vi "Logistic_Regression_with_iris_data.vi"() -> ()   [LabVIEW 2020]
doc: "Using logistic regression to classify the iris dataset."
uses:
  Model/Supervised/Linear_model/LinearClassifiers/LogisticRegression/Controls/logistic_regression_params.ctl
  Model/Supervised/Linear_model/LinearClassifiers/LogisticRegression/LogisticRegression.lvclass
  C:/Users/cipop/TDF Dropbox/2_Technologies de France/1 - Services et Etudes/PLAIY/2 - DEV/PLAIYLAB/code/Model/Model.lvclass
  Model/Supervised/Linear_model/LinearClassifiers/LogisticRegression/LogisticRegression.vi
panel:
  out "score":dbl
  out "y":dbl[][](array[numeric])
  in  "params":T1={"penalty"="l2", "dual"=FALSE, "tol"=0.0001, "C"=1.0, "fit_intercept"=FALSE, "intercept_scaling"=1.0, "class_weight"={"class_weight_type"="None", "class_weight_dict"=""}, "random_state"=0.0, "solver"="lbfgs", "max_iter"=100.0, "multi_class"="auto", "verbose"=0.0, "warm_start"=FALSE, "n_jobs"=1.0, "l1_ratio"={"l1_ratio_type"="None", "l1_ratio_float"=0.0}}
  out "XY Graph":T2(graph)
  out "error out":errorcluster
  out "X":dbl[][](array[numeric])
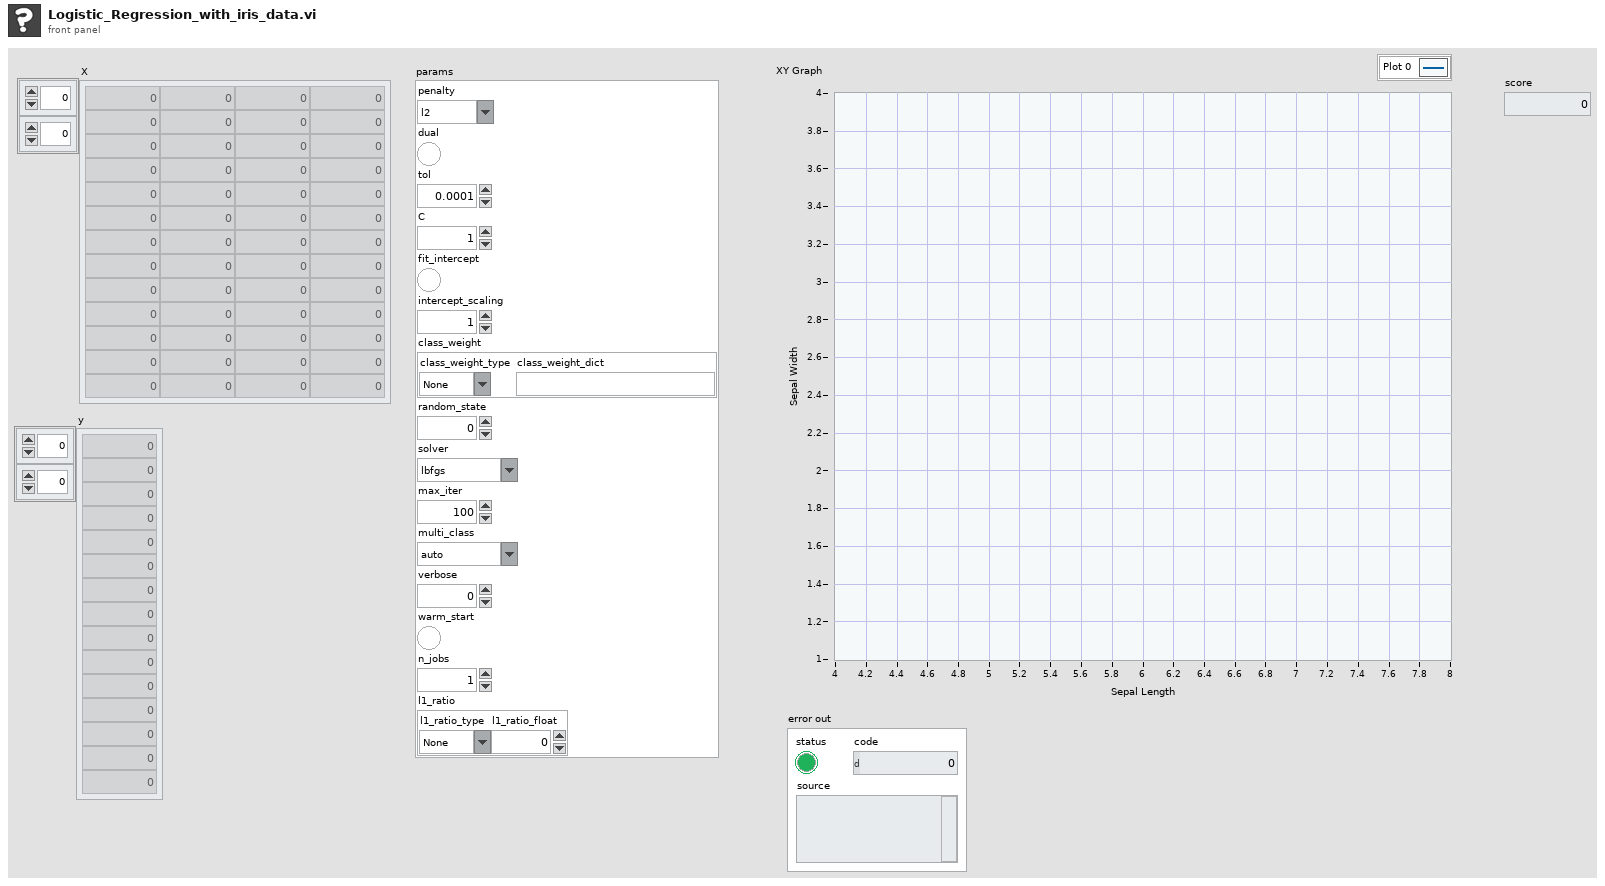
[diagram p1: front panel]
types:
  T1 = typedef "logistic_regression_params.ctl" = cluster{"penalty":string, "dual":bool, "tol":dbl, "C":dbl, "fit_intercept":bool, "intercept_scaling":dbl, "class_weight":cluster{"class_weight_type":string, "class_weight_dict":string}, "random_state":dbl, "solver":string, "max_iter":dbl, "multi_class":string, "verbose":dbl, "warm_start":bool, "n_jobs":dbl, "l1_ratio":cluster{"l1_ratio_type":string, "l1_ratio_float":dbl}}
  T2 = cluster{"XY Graph":cluster{"X":dbl, "Y":dbl}[]}[]
  T3 = cluster{"X Train":dbl[][], "X Test":dbl[][], "Y Train":dbl[][], "Y Test":dbl[][]}
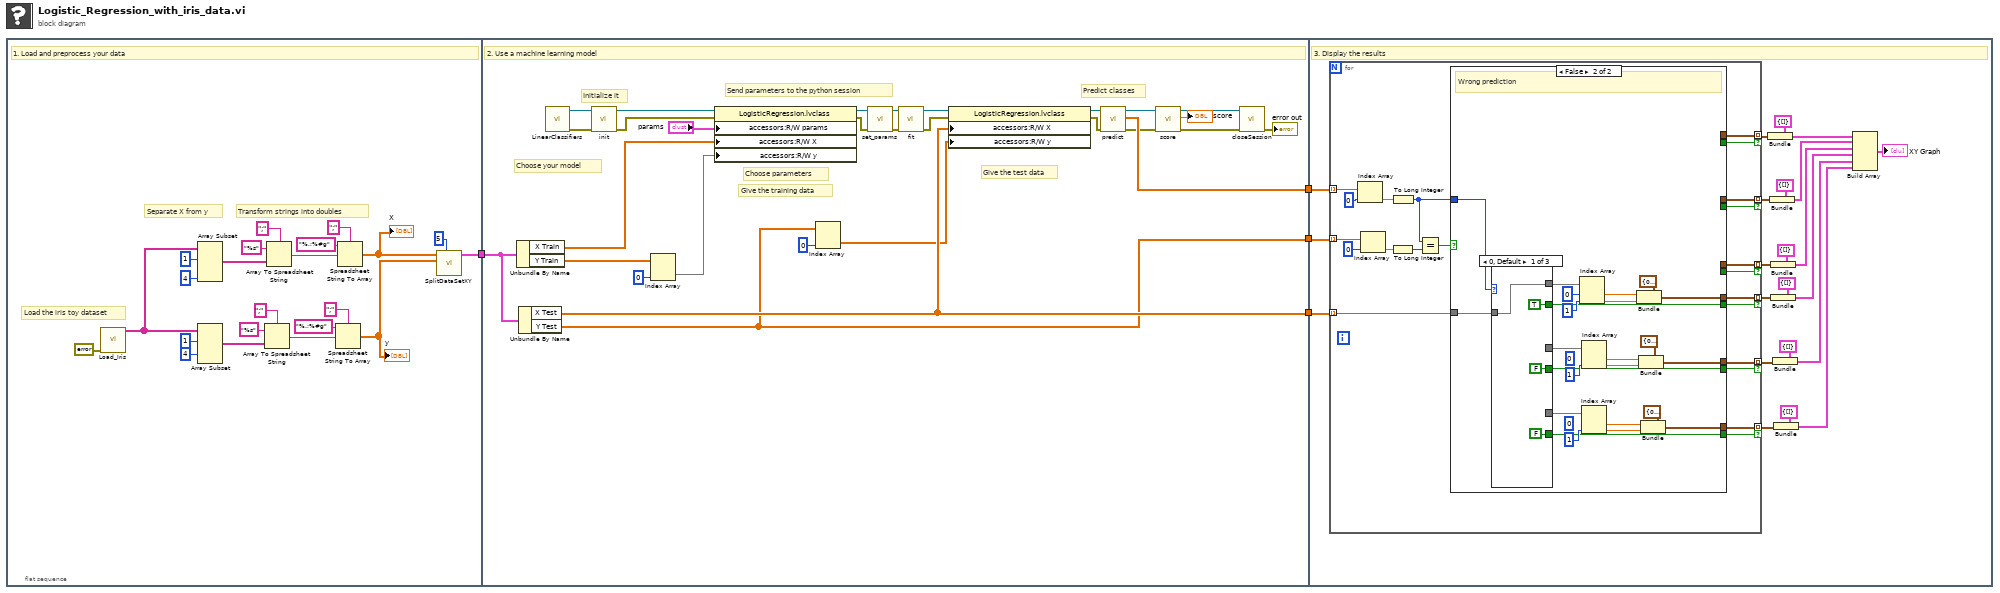
[diagram p0: block diagram]
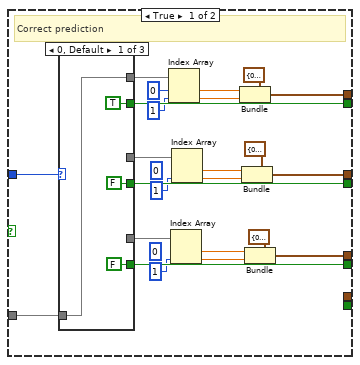
[diagram p2: hidden frame]
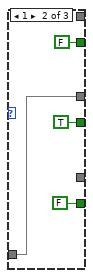
[diagram p3: hidden frame]
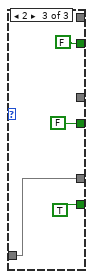
[diagram p4: hidden frame]
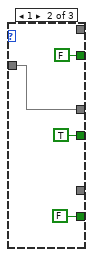
[diagram p5: hidden frame]
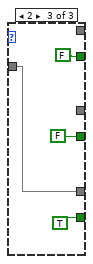
[diagram p6: hidden frame]
diagram:
  n1 = flat-sequence {
    tunnel: [w6] -> w2
    tunnel: [w47] -> w4
    tunnel: [w40] -> w3
    tunnel: w2 -> [w43]
    tunnel: [w33] -> w1
    tunnel: w4 -> [w76]
    tunnel: w3 -> [w77]
    tunnel: w1 -> [w65]
    frame #0 {
      # "Transform strings into doubles"
      # "Separate X from y"
      # "Load the iris toy dataset"
      # "1. Load and preprocess your data"
      n2 = call "Load_Iris.vi"("error in"=errorcluster {"status"=FALSE, "code"=0, "source"=""}) -> ("Tableau"=w21:string[][])  [unwired: 9 in, 1 out]
      n3 = Array Subset(array=w21, index (row)=1 ("index"), length (col)=4 ("length")) -> (w20:string[][])  [unwired: 2 in]
      n4 = Array Subset(array=w21, index (row)=1 ("index"), index (col)=4 ("index")) -> (w9:string[][])  [unwired: 2 in]
      n5 = Array To Spreadsheet String(delimiter (Tab)=";", array=w9, 3:"%s" ("format string")) -> (spreadsheet string=w10:string)
      n6 = Array To Spreadsheet String(delimiter (Tab)=";", array=w20, 3:"%s" ("format string")) -> (spreadsheet string=w15:string)
      n7 = Spreadsheet String To Array(delimiter (Tab)=";", format string="%.;%#g", spreadsheet string=w10) -> (array=w7:dbl[][])  [unwired: 1 in]
      "y" <- w7
      n8 = Spreadsheet String To Array(delimiter (Tab)=";", format string="%.;%#g", spreadsheet string=w15) -> (array=w8:dbl[][])  [unwired: 1 in]
      "X" <- w8
      n9 = call "SplitDataSetXY.vi"("%SplitTrain"=5, "Y"=w7, "X"=w8) -> ("Split"=w6:T3)  [unwired: 7 in, 1 out]
    }
    frame #1 {
      # "Predict classes"
      # "Give the test data"
      # "Send parameters to the python session"
      # "Give the training data"
      # "Choose parameters"
      # "Initialize it"
      # "Choose your model"
      # "2. Use a machine learning model"
      n10 = Unbundle By Name(w43) -> ("X Train"=w46:dbl[][], "Y Train"=w45:dbl[][])
      n11 = Unbundle By Name(w43) -> ("X Test"=w40:dbl[][], "Y Test"=w33:dbl[][])
      n12 = call-poly "LinearClassifiers.vi"() -> ("error out"=w31:errorcluster, "out"=w51:refnum<class "LogisticRegression.lvclass">)  [unwired: 10 in]
      n13 = call-dynamic "init.vi"("error in (no error)"=w31, "Model en entrée"=w51) -> ("error out"=w55:errorcluster, "Model en sortie"=w54:refnum<class "LogisticRegression.lvclass">)  [unwired: 8 in]
      n14 = Index Array(array=w45, index (col)=0 ("disabled index (col)")) -> (element=w44:dbl[])  [unwired: 1 in]
      n15 = property class="LogisticRegression.lvclass"(reference=w54, error in=w55, "accessors:R/W params"="params", "accessors:R/W X"=w46, "accessors:R/W y"=w44) -> (reference out=w53:refnum<class "LogisticRegression.lvclass">, error out=w52:errorcluster)
      n16 = Index Array(array=w33, index (col)=0 ("disabled index (col)")) -> (element=w32:dbl[])  [unwired: 1 in]
      n17 = call-dynamic "set_params.vi"("error in (no error)"=w52, "LogisticRegression.lvclass 2"=w53) -> ("error out"=w48:errorcluster, "LogisticRegression.lvclass"=w49:refnum<class "LogisticRegression.lvclass">)  [unwired: 8 in]
      n18 = call-dynamic "fit.vi"("error in (no error)"=w48, "LogisticRegression.lvclass 2"=w49) -> ("error out"=w41:errorcluster, "LogisticRegression.lvclass"=w42:refnum<class "LogisticRegression.lvclass">)  [unwired: 8 in]
      n19 = property class="LogisticRegression.lvclass"(reference=w42, error in=w41, "accessors:R/W X"=w40, "accessors:R/W y"=w32) -> (reference out=w38:refnum<class "LogisticRegression.lvclass">, error out=w39:errorcluster)
      n20 = call-dynamic "predict.vi"("error in (no error)"=w39, "LogisticRegression.lvclass 2"=w38) -> ("error out"=w35:errorcluster, "C"=w47:dbl[][], "LogisticRegression.lvclass"=w37:refnum<class "LogisticRegression.lvclass">)  [unwired: 7 in]
      n21 = call-dynamic "score.vi"("error in (no error)"=w35, "LogisticRegression.lvclass 2"=w37) -> ("error out"=w30:errorcluster, "score"=→"score":dbl, "LogisticRegression.lvclass"=w36:refnum<class "LogisticRegression.lvclass">)  [unwired: 7 in]
      n22 = call-dynamic "closeSession.vi"("error in"=w30, "Python en entrée"=w36) -> ("error out"=→"error out":errorcluster)  [unwired: 8 in, 1 out]
    }
    frame #2 {
      # "3. Display the results"
      n23 = for {
        tunnel: w77 -> [w96] mode=indexing
        tunnel: w76 -> [w99] mode=indexing
        tunnel: [w92] -> w74 mode=indexing if=w95
        tunnel: [w91] -> w72 mode=indexing if=w94
        tunnel: [w90] -> w70 mode=indexing if=w93
        tunnel: w65 -> [w87] mode=indexing
        tunnel: [w84] -> w61 mode=indexing if=w83
        tunnel: [w82] -> w60 mode=indexing if=w81
        tunnel: [w80] -> w59 mode=indexing if=w79
        n24 = Index Array(array=w99, index=0) -> (element=w97:dbl)
        n25 = Index Array(array=w87, index=0) -> (element=w88:dbl)
        n26 = To Long Integer(number=w88) -> (32bit integer=w85:i32)
        n27 = To Long Integer(number=w97) -> (32bit integer=w86:i32)
        n28 = Equal?(x=w86, y=w85) -> (x = y?=w78:bool)
        n29 = case shown="False" w78 {
          tunnel: w96 -> [w123 w159]
          tunnel: [w122 _] -> w95
          tunnel: [w121 _] -> w94
          tunnel: [w120 _] -> w93
          tunnel: [w103 _] -> w92
          tunnel: [w102 _] -> w91
          tunnel: [w101 _] -> w90
          tunnel: w86 -> [w100 w142]
          tunnel: [_ w141] -> w84
          tunnel: [_ w140] -> w83
          tunnel: [_ w139] -> w82
          tunnel: [_ w138] -> w81
          tunnel: [_ w137] -> w80
          tunnel: [_ w136] -> w79
          frame True {
            (unwired) 0 ("index")
            (unwired) 0 ("index")
            # "Correct prediction"
            n30 = case shown="0, Default" w100 {
              tunnel: w123 -> [w127 w130 w133]
              tunnel: [w127 _ _] -> w118
              tunnel: [TRUE FALSE FALSE] -> w122
              tunnel: [_ w130 _] -> w112
              tunnel: [FALSE TRUE FALSE] -> w121
              tunnel: [_ _ w133] -> w113
              tunnel: [FALSE FALSE TRUE] -> w120
              frame 0, Default {
              }
              frame 1 {
              }
              frame 2 {
              }
            }
            n31 = Index Array(array=w118, index #1=0 ("index"), index #2=1 ("index")) -> (element #1=w111:dbl, element #2=w110:dbl)
            n32 = Index Array(array=w113, index #2=1 ("index")) -> (element #1=w104:dbl, element #2=w105:dbl)  [unwired: 1 in]
            n33 = Index Array(array=w112, index #2=1 ("index")) -> (element #1=w107:dbl, element #2=w106:dbl)  [unwired: 1 in]
            n34 = Bundle(cluster=cluster{"X":dbl, "Y":dbl} {"X"=0.0, "Y"=0.0}, "X"=w111, "Y"=w110) -> (w103:cluster{"X":dbl, "Y":dbl})
            n35 = Bundle(cluster=cluster{"X":dbl, "Y":dbl} {"X"=0.0, "Y"=0.0}, "X"=w107, "Y"=w106) -> (w102:cluster{"X":dbl, "Y":dbl})
            n36 = Bundle(cluster=cluster{"X":dbl, "Y":dbl} {"X"=0.0, "Y"=0.0}, "X"=w104, "Y"=w105) -> (w101:cluster{"X":dbl, "Y":dbl})
          }
          frame False {
            (unwired) 0 ("index")
            (unwired) 0 ("index")
            # "Wrong prediction"
            n37 = case shown="0, Default" w142 {
              tunnel: w159 -> [w163 w166 w169]
              tunnel: [w163 _ _] -> w157
              tunnel: [TRUE FALSE FALSE] -> w140
              tunnel: [_ w166 _] -> w151
              tunnel: [FALSE TRUE FALSE] -> w138
              tunnel: [_ _ w169] -> w152
              tunnel: [FALSE FALSE TRUE] -> w136
              frame 0, Default {
              }
              frame 1 {
              }
              frame 2 {
              }
            }
            n38 = Index Array(array=w157, index #1=0 ("index"), index #2=1 ("index")) -> (element #1=w150:dbl, element #2=w149:dbl)
            n39 = Index Array(array=w152, index #2=1 ("index")) -> (element #1=w143:dbl, element #2=w144:dbl)  [unwired: 1 in]
            n40 = Index Array(array=w151, index #2=1 ("index")) -> (element #1=w146:dbl, element #2=w145:dbl)  [unwired: 1 in]
            n41 = Bundle(cluster=cluster{"X":dbl, "Y":dbl} {"X"=0.0, "Y"=0.0}, "X"=w150, "Y"=w149) -> (w141:cluster{"X":dbl, "Y":dbl})
            n42 = Bundle(cluster=cluster{"X":dbl, "Y":dbl} {"X"=0.0, "Y"=0.0}, "X"=w146, "Y"=w145) -> (w139:cluster{"X":dbl, "Y":dbl})
            n43 = Bundle(cluster=cluster{"X":dbl, "Y":dbl} {"X"=0.0, "Y"=0.0}, "X"=w143, "Y"=w144) -> (w137:cluster{"X":dbl, "Y":dbl})
          }
        }
      }
      n44 = Bundle(cluster=cluster{"XY Graph":cluster{"X":dbl, "Y":dbl}[]} {"XY Graph"=[]}, "XY Graph"=w74) -> (w69:cluster{"XY Graph":cluster{"X":dbl, "Y":dbl}[]})
      n45 = Bundle(cluster=cluster{"XY Graph":cluster{"X":dbl, "Y":dbl}[]} {"XY Graph"=[]}, "XY Graph"=w72) -> (w68:cluster{"XY Graph":cluster{"X":dbl, "Y":dbl}[]})
      n46 = Bundle(cluster=cluster{"XY Graph":cluster{"X":dbl, "Y":dbl}[]} {"XY Graph"=[]}, "XY Graph"=w70) -> (w67:cluster{"XY Graph":cluster{"X":dbl, "Y":dbl}[]})
      n47 = Bundle(cluster=cluster{"XY Graph":cluster{"X":dbl, "Y":dbl}[]} {"XY Graph"=[]}, "XY Graph"=w61) -> (w58:cluster{"XY Graph":cluster{"X":dbl, "Y":dbl}[]})
      n48 = Bundle(cluster=cluster{"XY Graph":cluster{"X":dbl, "Y":dbl}[]} {"XY Graph"=[]}, "XY Graph"=w60) -> (w57:cluster{"XY Graph":cluster{"X":dbl, "Y":dbl}[]})
      n49 = Bundle(cluster=cluster{"XY Graph":cluster{"X":dbl, "Y":dbl}[]} {"XY Graph"=[]}, "XY Graph"=w59) -> (w56:cluster{"XY Graph":cluster{"X":dbl, "Y":dbl}[]})
      n50 = Build Array(w69, w68, w67, w58, w57, w56) -> (→"XY Graph":T2)
    }
  }
